vi "NodeID to Channel Pointer.vi"(8 "error in (no error)":errorcluster, 11 "nodeID in":T1 format="%.0x") -> (0 "error out":errorcluster, 2 "BaseNodeType out":refnum<k24>, 3 "nodeID out":T1 format="%.0x")   [LabVIEW 2019, in "Instrument Addon Shared.lvlib"]
uses:
  Instrument Addon Shared.lvlib
  NationalInstruments.VeriStand.SystemDefinitionAPI
  <vilib>/NI VeriStand/Custom Device API/Custom Device Item Ref.ctl
  <vilib>/NI VeriStand/Custom Device API/Custom Device API.lvlib
  NationalInstruments.VeriStand.SystemStorage
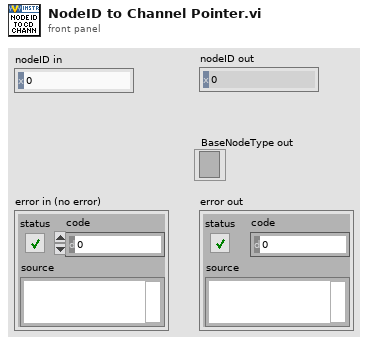
[diagram p1: front panel]
types:
  T1 = typedef "Custom Device API.lvlib/Custom Device Item Ref.ctl" = u64
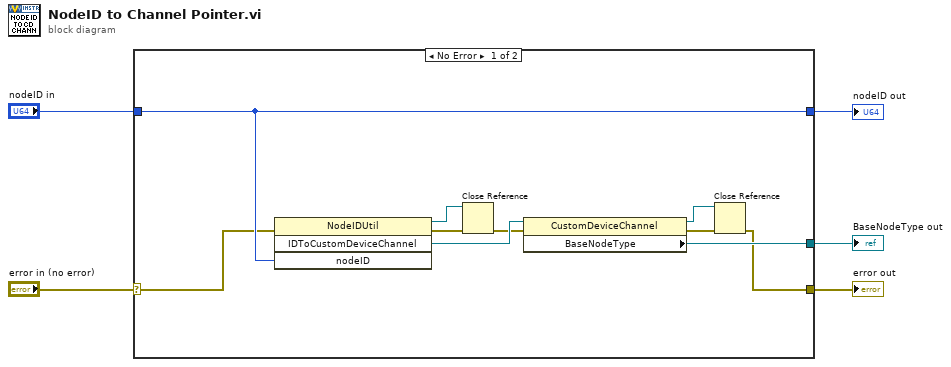
[diagram p0: block diagram]
diagram:
  n1 = case shown="No Error" "error in (no error)" {
    selector: "error in (no error)" -> [w9 w17]
    tunnel: "nodeID in" -> [w10 w16]
    tunnel: [w7 w17] -> w4
    tunnel: [w15 _] -> w3
    tunnel: [w10 w16] -> w2
    frame No Error {
      n2 = invoke class="NodeIDUtil" method="IDToCustomDeviceChannel"(error in=w9, "nodeID"=w10) -> (reference out=w12:refnum<k24>, error out=w13:errorcluster, "IDToCustomDeviceChannel"=w14:refnum<k24>)  [unwired: 2 in, 1 out]
      n3 = Close Reference(reference=w12, error in (no error)=w13) -> (error out=w11:errorcluster)
      n4 = property class="CustomDeviceChannel"(reference=w14, error in=w11) -> (reference out=w6:refnum<k24>, error out=w8:errorcluster, "BaseNodeType"=w15:refnum<k24>)
      n5 = Close Reference(reference=w6, error in (no error)=w8) -> (error out=w7:errorcluster)
    }
    frame Error {
    }
  }
  "error out" <- w4
  "BaseNodeType out" <- w3
  "nodeID out" <- w2
